vi "CloseProcess.vi"(8 "error in (no error)":errorcluster, 10 "ms timeout (1000)":i32=1000, 11 "obj":refnum<class "SimPump.lvclass">) -> (0 "error out":errorcluster, 3 "obj out":refnum<class "SimPump.lvclass">)   [LabVIEW 2019, in "SimPump.lvclass"]
doc: "Closes the active object process.\n\nwww.sciware.com.au"
uses:
  SimPump.lvclass
  MsgQueueType.ctl
  SimPump.lvclass/SimPump.ctl
panel:
  # "BSD License (http://www.opensource.org/licenses/bsd-license.php)"
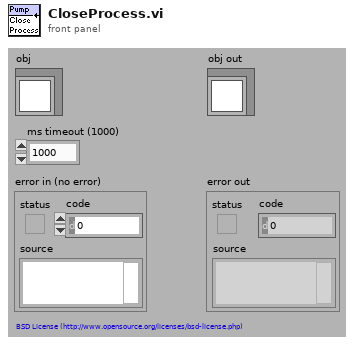
[diagram p1: front panel]
types:
  T1 = typedef "SimPump.lvclass/MsgQueueType.ctl" = string
  T2 = typedef "SimPump.lvclass/MsgQueueRef.ctl" = refnum<queue>
  T3 = typedef "SimPump.lvclass/CmdQueueRef.ctl" = refnum<queue>
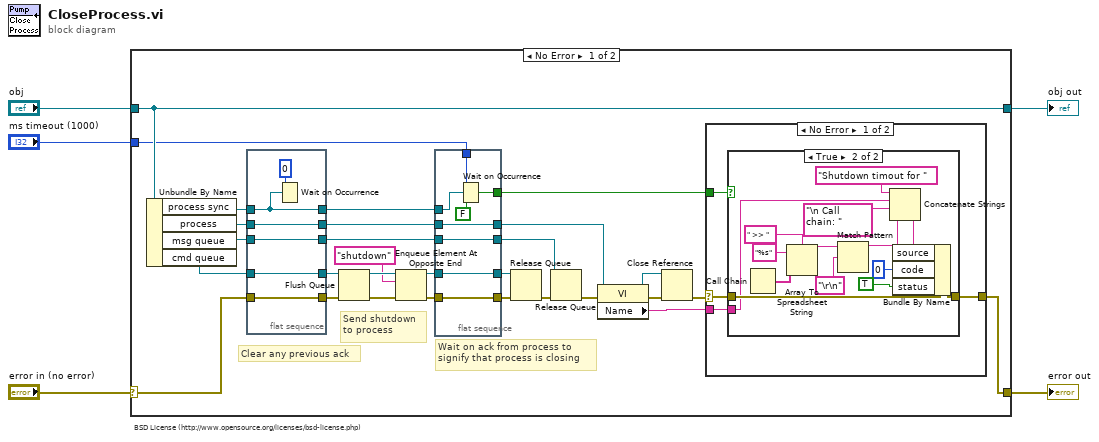
[diagram p0: block diagram]
diagram:
  # "BSD License (http://www.opensource.org/licenses/bsd-license.php)"
  n1 = case shown="No Error" "error in (no error)" {
    selector: "error in (no error)" -> [w30 w70]
    tunnel: [w17 w70] -> w4
    tunnel: [w34 w69] -> w2
    tunnel: "obj" -> [w34 w69]
    tunnel: "ms timeout (1000)" -> [w19 _]
    frame No Error {
      # "Send shutdown\nto process"
      # "Wait on ack from process to\nsignify that process is closing"
      # "Clear any previous ack"
      n2 = Unbundle By Name(w34) -> ("process sync"=w25:refnum<k4>, "process"=w27:refnum<vi>, "msg queue"=w8:T2, "cmd queue"=w9:T3)
      n3 = flat-sequence {
        tunnel: w30 -> [w60]
        tunnel: [w60] -> w29
        tunnel: [w59] -> w28
        tunnel: w9 -> [w59]
        tunnel: [w58] -> w26
        tunnel: w27 -> [w58]
        tunnel: w25 -> [w57]
        tunnel: [w57] -> w24
        tunnel: [w55] -> w7
        tunnel: w8 -> [w55]
        frame #0 {
          n4 = Wait on Occurrence(2:w57, 3:0 ("ms timeout (-1)")) -> ()  [unwired: 1 in, 1 out]
        }
      }
      n5 = Flush Queue(queue=w28, error in (no error)=w29) -> (queue out=w32:T3, error out=w33:errorcluster)  [unwired: 1 out]
      n6 = Enqueue Element At Opposite End(queue=w32, element=T1 "shutdown", error in (no error)=w33) -> (queue out=w23:T3, error out=w31:errorcluster)  [unwired: 1 in, 1 out]
      n7 = flat-sequence {
        tunnel: w31 -> [w68]
        tunnel: [w68] -> w22
        tunnel: w24 -> [w67]
        tunnel: [w66] -> w12
        tunnel: w26 -> [w66]
        tunnel: [w64] -> w21
        tunnel: w23 -> [w64]
        tunnel: w19 -> [w63]
        tunnel: [w62] -> w16
        tunnel: [w61] -> w6
        tunnel: w7 -> [w61]
        frame #0 {
          n8 = Wait on Occurrence(1:FALSE ("ignore previous (T)"), 2:w67, 3:w63) -> (0:w62:bool)
        }
      }
      n9 = Release Queue(queue=w21, error in (no error)=w22) -> (error out=w20:errorcluster)  [unwired: 1 in, 2 out]
      n10 = Release Queue(queue=w6, error in (no error)=w20) -> (error out=w15:errorcluster)  [unwired: 1 in, 2 out]
      n11 = property class="VI"(reference=w12, error in=w15) -> (reference out=w13:refnum<vi>, error out=w14:errorcluster, "Name"=w11:string)
      n12 = Close Reference(reference=w13, error in (no error)=w14) -> (error out=w18:errorcluster)
      n13 = case shown="No Error" w18 {
        selector: w18 -> [w38 w54]
        tunnel: [w37 w54] -> w17
        tunnel: w16 -> [w36 _]
        tunnel: w11 -> [w35 _]
        frame No Error {
          n14 = case shown="True" w36 {
            tunnel: w38 -> [w39 w42]
            tunnel: [w39 w41] -> w37
            tunnel: w35 -> [_ w40]
            frame False {
            }
            frame True {
              n15 = Call Chain() -> (call chain=w46:string[])
              n16 = Array To Spreadsheet String(delimiter (Tab)=" >> ", array=w46, 3:"%s" ("format string")) -> (spreadsheet string=w47:string)
              n17 = Match Pattern(string=w47, regular expression="\r\n") -> (before substring=w45:string)  [unwired: 4 out]
              n18 = Concatenate Strings("Shutdown timout for " ("source"), w40, "\n Call chain: " ("string"), w45) -> (w53:string)
              n19 = Bundle By Name(cluster=w42, "source"=w53, "code"=0, "status"=TRUE) -> (w41:errorcluster)
            }
          }
        }
        frame Error {
        }
      }
    }
    frame Error {
    }
  }
  "error out" <- w4
  "obj out" <- w2
